vi "Do.vi"(8 "error in":errorcluster, 10 "Actor in":refnum<class "Actor.lvclass">, 11 "Start Calibration MSG":refnum<class "Start Calibration MSG.lvclass">) -> (0 "error out":errorcluster, 2 "Actor out":refnum<class "Actor.lvclass">)   [LabVIEW 2018, in "Controller.lvlib" / "Start Calibration MSG.lvclass"]
doc: "(<B>Filename</B>: Actor Framework.lvlib:Message.lvclass:Do.vi)\n\nDefines what a message does when it is received by an actor. Generally, a message instructs an actor to invoke one of its methods. By default, this method does nothing. A child class must override it to define behavior. Create a child class by using the Actor Framework Message Maker dialog box."
uses:
  Start Calibration MSG.lvclass
  <vilib>/ActorFramework/Actor/Actor.lvclass
  Start Calibration MSG.lvclass/Start Calibration MSG.ctl
  Calibration/Actor/Calibration Actor.lvclass
  C:/Users/Labview/Documents/exscalabar_server/SuperActor/SuperActor.lvclass
  C:/Program Files (x86)/National Instruments/LabVIEW 2018/vi.lib/ActorFramework/Actor/Actor.lvclass
  Controller.lvclass
  Calibration/Actor/Calibration Actor.lvclass/Calibration Actor.ctl
  SuperActor/SuperActor.lvclass/SuperActor.ctl
  Calibration/Actor/Write CalPath.vi
  SuperActor/Write ID.vi
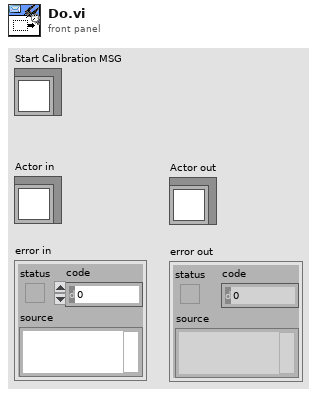
[diagram p1: front panel]
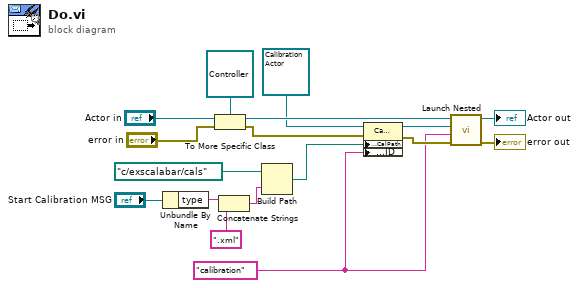
[diagram p0: block diagram]
diagram:
  w1 = "calibration" ("ID")
  n1 = Unbundle By Name("Start Calibration MSG") -> ("type"=w10:string)
  n2 = To More Specific Class(target class=refnum<class "Controller.lvclass"> refnum ("Controller:Controller"), reference="Actor in", error in="error in") -> (specific class reference=w15:refnum<class "Controller.lvclass">, error out=w3:errorcluster)
  n3 = Concatenate Strings(w10, ".xml" ("string")) -> (w8:string)
  n4 = Build Path(base path=path "c:/exscalabar/cals", name or relative path=w8) -> (appended path=w6:path)
  n5 = property class="Calibration Actor"(reference=refnum<class "Calibration Actor.lvclass"> refnum ("Calibration.lvlib:Calibration Actor"), error in=w3, "Accessors:CalPath"=w6, "Accessors:ID"=w1) -> (reference out=w5:refnum<class "Calibration Actor.lvclass">, error out=w4:errorcluster)
  n6 = call "Launch Nested.vi"("Error In"=w4, "ID"=w1, "Nested Actor"=w5, "Controller in"=w15) -> ("Error Out"=→"error out":errorcluster, "Controller out"=→"Actor out":refnum<class "Controller.lvclass">)  [unwired: 4 in, 2 out]
